vi "high_res_delay.vi"(8 "error in (no error)":errorcluster, 11 "Delay (sec)":dbl format="%#_13g") -> (0 "error out":errorcluster)   [LabVIEW 2011]
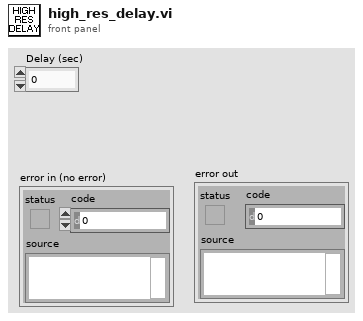
[diagram p1: front panel]
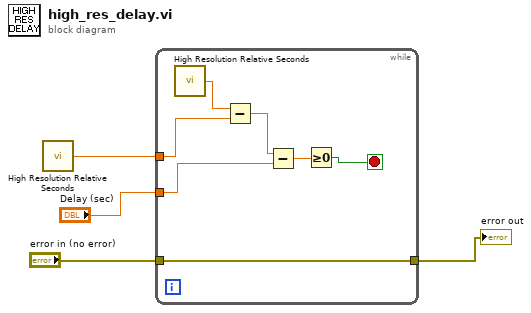
[diagram p0: block diagram]
diagram:
  n1 = call <vilib>:"High Resolution Relative Seconds.vi"() -> ("relative seconds"=w4:dbl)
  n2 = while {
    tunnel: w4 -> [w10]
    tunnel: "Delay (sec)" -> [w7]
    tunnel: [w5] -> w2
    tunnel: "error in (no error)" -> [w5]
    stop <- w6 stop-if-true
    n3 = call <vilib>:"High Resolution Relative Seconds.vi"() -> ("relative seconds"=w11:dbl)
    n4 = Subtract(x=w11, y=w10) -> (x-y=w8:dbl)
    n5 = Subtract(x=w8, y=w7) -> (x-y=w9:dbl)
    n6 = Greater Or Equal To 0?(x=w9) -> (x >= 0?=w6:bool)
  }
  "error out" <- w2
